vi "Create Template Sech2 Function.vi"(10 "w":dbl, 11 "N":dbl) -> (3 "Array":dbl[](array[numeric]))   [LabVIEW 2016]
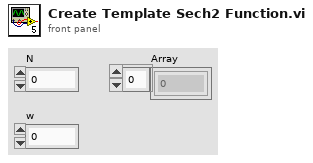
[diagram p1: front panel]
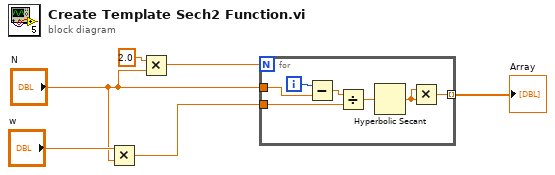
[diagram p0: block diagram]
diagram:
  n1 = Multiply(x="w", y="N") -> (x*y=w2:dbl)
  n2 = Multiply(x=2.0, y="N") -> (x*y=w4:dbl)
  n3 = for {
    N: w4 -> [_]
    tunnel: "N" -> [w12]
    tunnel: w2 -> [w10]
    tunnel: [w7] -> w6 mode=indexing
    i -> [w13]
    n4 = Subtract(x=w13, y=w12) -> (x-y=w11:dbl)
    n5 = Divide(x=w11, y=w10) -> (x/y=w9:dbl)
    n6 = Hyperbolic Secant(1:w9) -> (0:w8:dbl)
    n7 = Multiply(x=w8, y=w8) -> (x*y=w7:dbl)
  }
  "Array" <- w6
